vi "Generate Service Config JSON.vi"(0 "display name":string, 1 "description URL":string, 5 "service class":string, 7 "provided interfaces":string[](array[string]), 9 "path":string, 11 "error in":errorcluster, 12 "annotations":T1[](array[typedef])) -> (4 "service config JSON":string, 15 "error out":errorcluster)   [LabVIEW 2020, in "Plug-In SDK Measurement.lvlib"]
uses:
  Plug-In SDK Measurement.lvlib
  TypeDefs/Measurement Annotation.ctl
  867c5996-9fc4-446f-bc7e-cd1af3184270.vi
  a066e80c-61f1-4c64-8e78-6e3d97fd6b7b.vi
  2858ca83-f95f-4d85-8bb1-5ba8a53c7693.vi
  26abaa1b-7193-4077-a3e4-3b2bfa2f984b.vi
  b2866af8-bc70-4c0d-b595-9f5224cfa858.vi
  0c37daab-07df-4eb5-bca5-1a967d50c5e0.vi
  867c5996-9fc4-446f-bc7e-cd1af3184270.vi/49d2641b-58d2-418d-86ef-5c98235809e6.vi
  867c5996-9fc4-446f-bc7e-cd1af3184270.vi/729eb87d-9ab4-481c-bd0a-7090d6acb718.vi
  a066e80c-61f1-4c64-8e78-6e3d97fd6b7b.vi/49d2641b-58d2-418d-86ef-5c98235809e6.vi
  a066e80c-61f1-4c64-8e78-6e3d97fd6b7b.vi/729eb87d-9ab4-481c-bd0a-7090d6acb718.vi
  2858ca83-f95f-4d85-8bb1-5ba8a53c7693.vi/49d2641b-58d2-418d-86ef-5c98235809e6.vi
  2858ca83-f95f-4d85-8bb1-5ba8a53c7693.vi/729eb87d-9ab4-481c-bd0a-7090d6acb718.vi
  26abaa1b-7193-4077-a3e4-3b2bfa2f984b.vi/49d2641b-58d2-418d-86ef-5c98235809e6.vi
  26abaa1b-7193-4077-a3e4-3b2bfa2f984b.vi/729eb87d-9ab4-481c-bd0a-7090d6acb718.vi
  b2866af8-bc70-4c0d-b595-9f5224cfa858.vi/49d2641b-58d2-418d-86ef-5c98235809e6.vi
  b2866af8-bc70-4c0d-b595-9f5224cfa858.vi/729eb87d-9ab4-481c-bd0a-7090d6acb718.vi
  0c37daab-07df-4eb5-bca5-1a967d50c5e0.vi/49d2641b-58d2-418d-86ef-5c98235809e6.vi
  0c37daab-07df-4eb5-bca5-1a967d50c5e0.vi/729eb87d-9ab4-481c-bd0a-7090d6acb718.vi
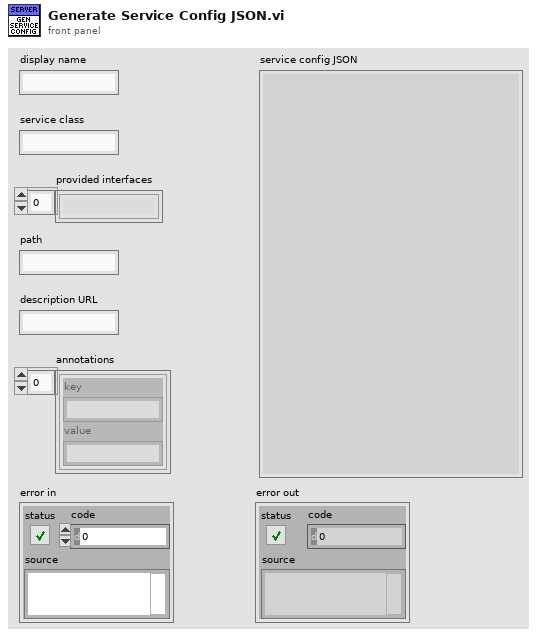
[diagram p1: front panel]
types:
  T1 = typedef "Plug-In SDK Measurement.lvlib/Measurement Annotation.ctl" = cluster{"key":string, "value":string}
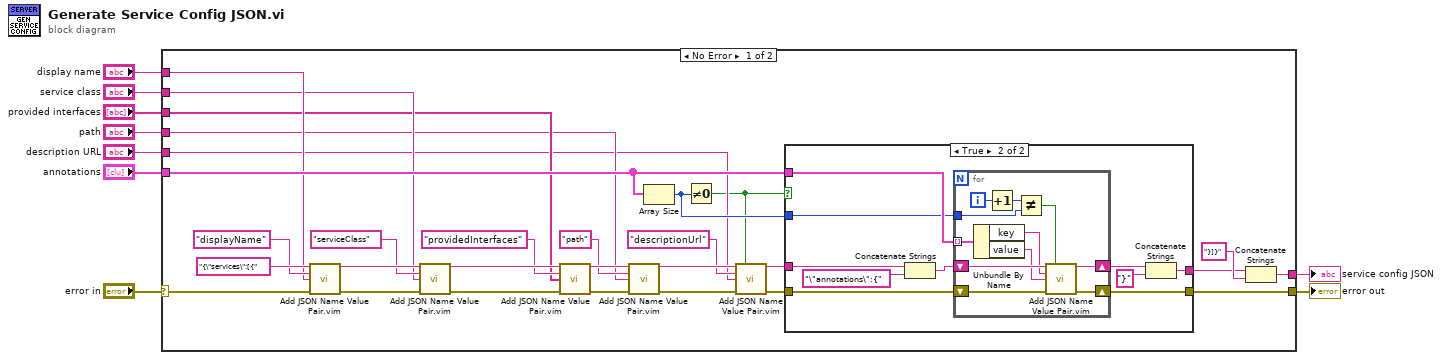
[diagram p0: block diagram]
diagram:
  n1 = case shown="No Error" "error in" {
    selector: "error in" -> [w32 w62]
    tunnel: [w36 w62] -> w8
    tunnel: "display name" -> [w29 _]
    tunnel: "service class" -> [w25 _]
    tunnel: "provided interfaces" -> [w21 _]
    tunnel: [w37 _] -> w4
    tunnel: "path" -> [w17 _]
    tunnel: "description URL" -> [w12 _]
    tunnel: "annotations" -> [w35 _]
    frame No Error {
      n2 = call "Add JSON Name Value Pair.vim"("JSON string in"="{\"services\":[{", "name"="displayName", "value"=w29, "error in"=w32) -> ("JSON string out"=w27:string, "error out"=w28:errorcluster)  [unwired: 10 in]
      n3 = call "Add JSON Name Value Pair.vim"("JSON string in"=w27, "name"="serviceClass", "value"=w25, "error in"=w28) -> ("JSON string out"=w23:string, "error out"=w24:errorcluster)  [unwired: 10 in]
      n4 = call "Add JSON Name Value Pair.vim"("JSON string in"=w23, "name"="providedInterfaces", "value"=w21, "error in"=w24) -> ("JSON string out"=w19:string, "error out"=w20:errorcluster)  [unwired: 10 in]
      n5 = call "Add JSON Name Value Pair.vim"("JSON string in"=w19, "name"="path", "value"=w17, "error in"=w20) -> ("JSON string out"=w14:string, "error out"=w16:errorcluster)  [unwired: 10 in]
      n6 = Array Size(array=w35) -> (size(s)=w34:i32)
      n7 = Not Equal To 0?(x=w34) -> (x != 0?=w11:bool)
      n8 = call "Add JSON Name Value Pair.vim"("JSON string in"=w14, "include trailing comma"=w11, "name"="descriptionUrl", "value"=w12, "error in"=w16) -> ("JSON string out"=w10:string, "error out"=w15:errorcluster)  [unwired: 9 in]
      n9 = case shown="True" w11 {
        tunnel: w15 -> [w40 w50]
        tunnel: [w40 w49] -> w36
        tunnel: w35 -> [_ w48]
        tunnel: w34 -> [_ w45]
        tunnel: [w39 w42] -> w33
        tunnel: w10 -> [w39 w41]
        frame False {
        }
        frame True {
          n10 = Concatenate Strings(w41, "\"annotations\":{") -> (w46:string)
          n11 = for {
            shift-right: [w56] -> w49
            shift-left: w50 -> [w57]
            tunnel: w48 -> [w59] mode=indexing
            shift-right: [w54] -> w44
            shift-left: w46 -> [w55]
            tunnel: w45 -> [w58]
            i -> [w61]
            n12 = Unbundle By Name(w59) -> ("key"=w51:string, "value"=w52:string)
            n13 = Increment(x=w61) -> (x+1=w60:i32)
            n14 = Not Equal?(x=w60, y=w58) -> (x != y?=w53:bool)
            n15 = call "Add JSON Name Value Pair.vim"("JSON string in"=w55, "include trailing comma"=w53, "name"=w51, "value"=w52, "error in"=w57) -> ("JSON string out"=w54:string, "error out"=w56:errorcluster)  [unwired: 9 in]
          }
          n16 = Concatenate Strings(w44, "}") -> (w42:string)
        }
      }
      n17 = Concatenate Strings(w33, "}]}") -> (w37:string)
    }
    frame Error {
    }
  }
  "error out" <- w8
  "service config JSON" <- w4
